vi "力特性 分离数据.vi"(9 "油压":dbl[](array[numeric]), 11 "扭矩":dbl[](array[numeric])) -> (0 "油压正转回":dbl[](array[numeric]), 1 "油压正转去":dbl[](array[numeric]), 2 "扭矩反转回":dbl[](array[numeric]), 3 "扭矩反转去":dbl[](array[numeric]), 4 "油压反转去":dbl[](array[numeric]), 5 "扭矩正转回":dbl[](array[numeric]), 6 "油压反转回":dbl[](array[numeric]), 7 "扭矩正转去":dbl[](array[numeric]))   [LabVIEW 2015, in "Logging.lvlib"]
uses:
  Logging.lvlib
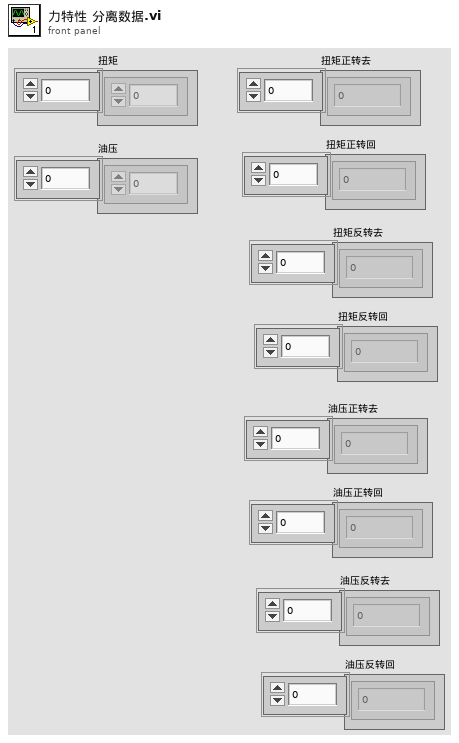
[diagram p1: front panel]
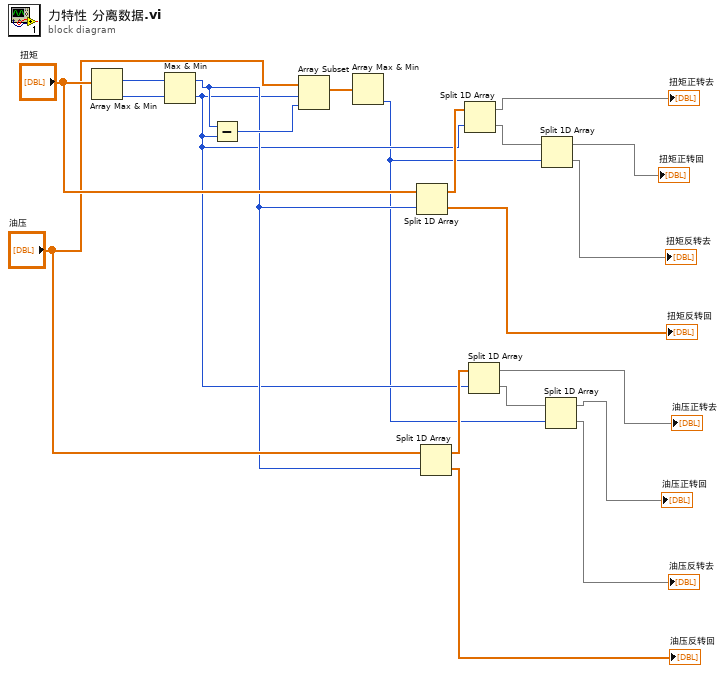
[diagram p0: block diagram]
diagram:
  n1 = Array Max & Min(array="扭矩") -> (max index (indices)=w21:i32, min index (indices)=w20:i32)  [unwired: 2 out]
  n2 = Max & Min(x=w21, y=w20) -> (max(x,y)=w7:i32, min(x,y)=w6:i32)
  n3 = Subtract(x=w7, y=w6) -> (x-y=w17:i32)
  n4 = Array Subset(array="油压", index=w6, length=w17) -> (w16:dbl[])
  n5 = Array Max & Min(array=w16) -> (min index (indices)=w5:i32)  [unwired: 3 out]
  n6 = Split 1D Array(array="扭矩", index=w7) -> (first subarray=w18:dbl[], second subarray=→"扭矩反转回":dbl[])
  n7 = Split 1D Array(array="油压", index=w7) -> (first subarray=w10:dbl[], second subarray=→"油压反转回":dbl[])
  n8 = Split 1D Array(array=w18, index=w6) -> (first subarray=→"扭矩正转去":dbl[], second subarray=w15:dbl[])
  n9 = Split 1D Array(array=w10, index=w6) -> (first subarray=→"油压正转去":dbl[], second subarray=w9:dbl[])
  n10 = Split 1D Array(array=w15, index=w5) -> (first subarray=→"扭矩正转回":dbl[], second subarray=→"扭矩反转去":dbl[])
  n11 = Split 1D Array(array=w9, index=w5) -> (first subarray=→"油压正转回":dbl[], second subarray=→"油压反转去":dbl[])
